vi "Reclose Virtual Relays.vi"(8 "error in (no error)":errorcluster, 9 "Relay Count Subarray [Count>0] In":i32[](array[numeric]), 11 "SLSC Switch in":refnum<class "SLSC Switch.lvclass">) -> (0 "error out":errorcluster, 3 "SLSC Switch out":refnum<class "SLSC Switch.lvclass">)   [LabVIEW 2016, in "SLSC Switch.lvlib" / "SLSC Switch.lvclass"]
doc: "Recloses the shared relays that were opened when the DLL Disconnect function was executed"
uses:
  SLSC Switch.lvclass
  SLSC Switch.lvclass/SLSC Switch.ctl
  slscsl/RelayAction.ctl
  Relay/Relay.lvclass/Relay.ctl
  Switch Action Processor/Switch Action Processor.lvclass
  slscsl/slscsl.lvclass
  Relay/Relay.lvclass
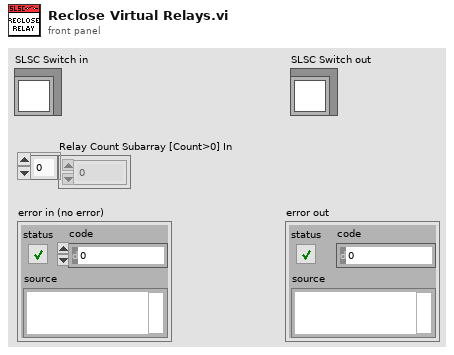
[diagram p1: front panel]
types:
  T1 = typedef "SLSC Switch.lvlib/slscsl.lvclass/RelayAction.ctl" = u32
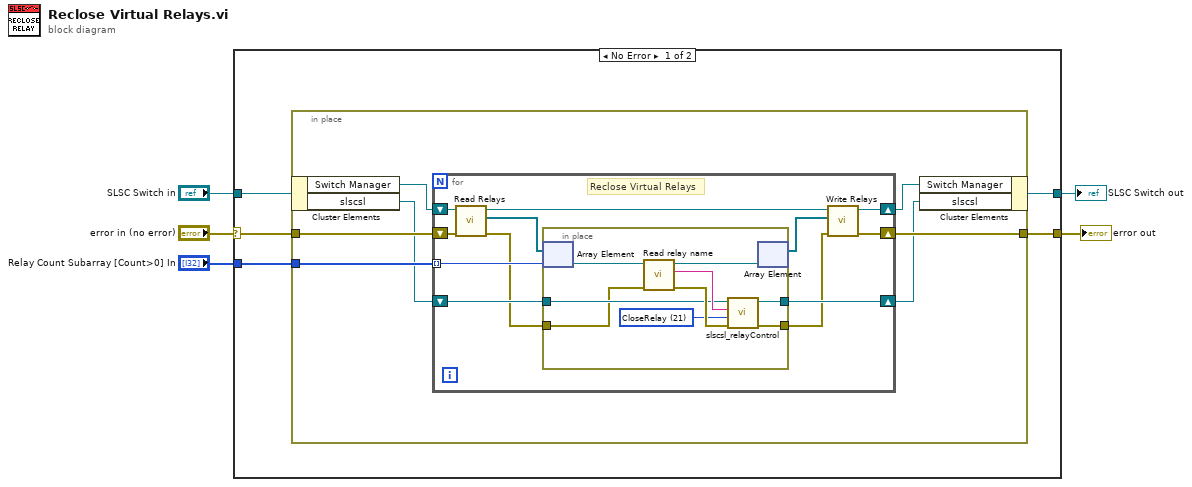
[diagram p0: block diagram]
diagram:
  n1 = case shown="No Error" "error in (no error)" {
    selector: "error in (no error)" -> [w8 w40]
    tunnel: "Relay Count Subarray [Count>0] In" -> [w10 _]
    tunnel: [w9 w40] -> w4
    tunnel: "SLSC Switch in" -> [w7 w39]
    tunnel: [w6 w39] -> w1
    frame No Error {
      n2 = in-place {
        in-place-border: w10 -> [w17]
        in-place-border: [w16] -> w9
        in-place-border: w8 -> [w15]
        n3 = in-place-cluster #1(w7) -> ("Switch Manager"=w14:refnum<class "Switch Action Processor.lvclass">, "slscsl"=w13:refnum<class "slscsl.lvclass">)
        n4 = for {
          shift-right: [w28] -> w11
          shift-left: w13 -> [w29]
          shift-right: [w26] -> w16
          shift-left: w15 -> [w18]
          tunnel: w17 -> [w25] mode=indexing
          shift-right: [w23] -> w12
          shift-left: w14 -> [w22]
          # "Reclose Virtual Relays"
          n5 = call-dynamic "Read Relays.vi"("error in (no error)"=w18, "Switch Action Processor in"=w22) -> ("error out"=w19:errorcluster, "Relays"=w20:refnum<class "Relay.lvclass">[], "Switch Action Processor out"=w21:refnum<class "Switch Action Processor.lvclass">)  [unwired: 7 in]
          n6 = in-place {
            in-place-border: w29 -> [w34]
            in-place-border: [w33] -> w28
            in-place-border: w19 -> [w32]
            in-place-border: [w30] -> w27
            w37 = T1 21 items=["CloseRelay"=21, "OpenRelay"=20] ("RelayAction")
            n7 = in-place-array #2(w20, w25) -> (w35:refnum<class "Relay.lvclass">)
            n8 = call "Read relay name.vi"("error in (no error)"=w32, "Relay in"=w35) -> ("error out"=w38:errorcluster, "name"=w36:string, "Relay out"=w31:refnum<class "Relay.lvclass">)  [unwired: 7 in]
            n9 = call "slscsl_relayControl.vi"("error in (no error)"=w38, "RelayAction"=w37, "relayNames"=w36, "slscsl in"=w34) -> ("error out"=w30:errorcluster, "slscsl out"=w33:refnum<class "slscsl.lvclass">)  [unwired: 5 in, 1 out]
            n10 = in-place-array #2(w31) -> (w24:refnum<class "Relay.lvclass">[])  [unwired: 1 out]
          }
          n11 = call-dynamic "Write Relays.vi"("error in (no error)"=w27, "Relays"=w24, "Switch Action Processor in"=w21) -> ("error out"=w26:errorcluster, "Switch Action Processor out"=w23:refnum<class "Switch Action Processor.lvclass">)  [unwired: 7 in]
        }
        n12 = in-place-cluster #1("Switch Manager"=w12, "slscsl"=w11) -> (w6:refnum<class "SLSC Switch.lvclass">)
      }
    }
    frame Error {
    }
  }
  "error out" <- w4
  "SLSC Switch out" <- w1
